vi "Init Data.vi"(10 "Data":T1) -> (3 "Msg out":refnum<class "Msg.lvclass">)   [LabVIEW 2020, in "Event.lvlib" / "Msg.lvclass"]
uses:
  Msg.lvclass
  Data.ctl
  EventLevel/Enumeration.ctl
  Error/Data.ctl
  Msg.lvclass/Msg.ctl
  Event.lvlib
  Error/Error.lvlib
  EventLevel/EventLevel.lvlib
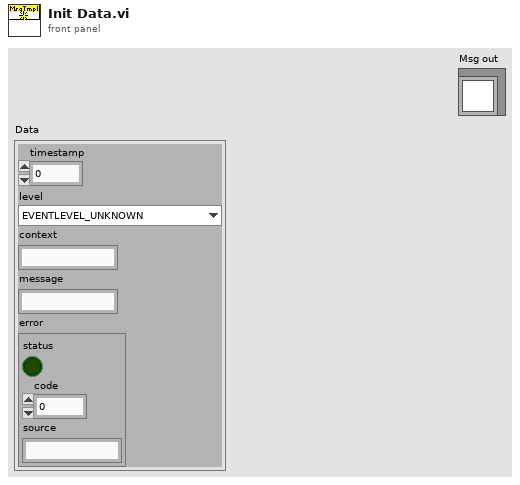
[diagram p1: front panel]
types:
  T1 = typedef "Event.lvlib/Data.ctl" = cluster{"timestamp":i64, "level":T2, "context":string, "message":string, "error":T3}
  T2 = typedef "EventLevel.lvlib/Enumeration.ctl" = enum16{"EVENTLEVEL_UNKNOWN", "EVENTLEVEL_DEBUG", "EVENTLEVEL_INFO", "EVENTLEVEL_WARNING", "EVENTLEVEL_ERROR"}
  T3 = typedef "Error.lvlib/Data.ctl" = errorcluster
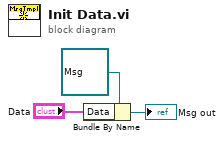
[diagram p0: block diagram]
diagram:
  n1 = Bundle By Name(cluster=refnum<class "Msg.lvclass"> refnum ("Msg out"), "Data"="Data") -> (→"Msg out":refnum<class "Msg.lvclass">)
